vi "Get pin Status.vi"(8 "error in (no error)":errorcluster, 9 "Pin 2":dbl, 10 "Puerto":dbl, 11 "Simulado in":refnum<class "Simulado.lvclass">) -> (0 "error out":errorcluster, 3 "Simulado out":refnum<class "Simulado.lvclass">)   [LabVIEW 2020, in "Simulado.lvclass"]
uses:
  Simulado.lvclass
  Simulado.lvclass/Simulado.ctl
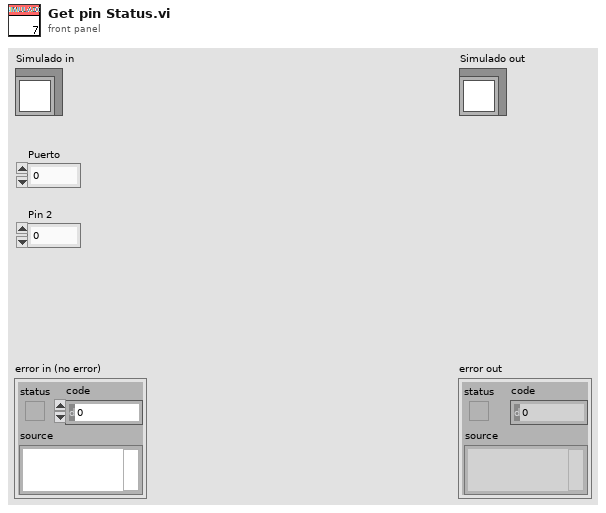
[diagram p1: front panel]
types:
  T1 = typedef "Serial Device.lvclass/serial device brand.ctl" = string
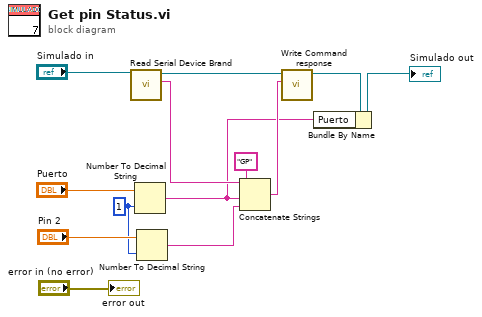
[diagram p0: block diagram]
diagram:
  w9 = i16 1 ("width (-)")
  n1 = call-dynamic "Read Serial Device Brand.vi"("Serial Device in"="Simulado in") -> ("Serial Device Brand"=w8:T1, "Serial Device out"=w12:refnum<class "Simulado.lvclass">)  [unwired: 8 in, 1 out]
  n2 = Number To Decimal String(number="Puerto", width (-)=w9) -> (decimal integer string=w1:string)
  n3 = Number To Decimal String(number="Pin 2", width (-)=w9) -> (decimal integer string=w6:string)
  n4 = Concatenate Strings(w8, "GP" ("string"), w1, w6) -> (w2:string)
  n5 = call-dynamic "Write Command response.vi"("Command response"=w2, "Simulado in"=w12) -> ("Simulado out"=w5:refnum<class "Simulado.lvclass">)  [unwired: 8 in, 1 out]
  n6 = Bundle By Name(cluster=w5, "Puerto"=w1) -> (→"Simulado out":refnum<class "Simulado.lvclass">)
  "error out" <- "error in (no error)"
